vi "myRIO_BRig_Host_parse_dataTrial__read__compare.vi"(8 "input_arrayCtrl":i32[][](array[numeric]), 9 "input_idxCtrl":i32, 10 "input_arraySample":i32[][](array[numeric]), 11 "input_idxSample":i32) -> (2 "output_arraySample":i32[][](array[numeric]), 3 "output_idxSample":i32)   [LabVIEW 2014]
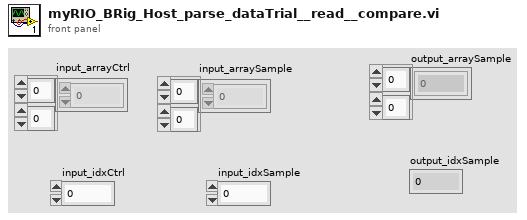
[diagram p1: front panel]
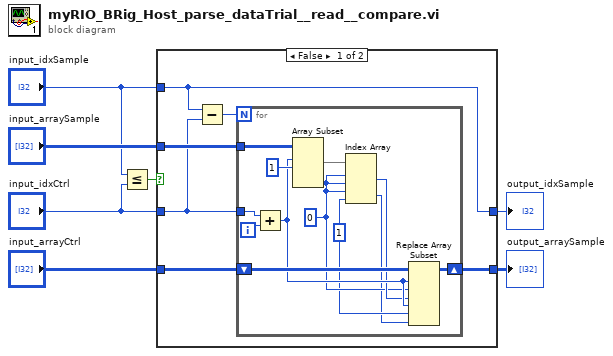
[diagram p0: block diagram]
diagram:
  n1 = Less Or Equal?(x="input_idxSample", y="input_idxCtrl") -> (x <= y?=w7:bool)
  n2 = case shown="False" w7 {
    tunnel: "input_arrayCtrl" -> [w11 w27]
    tunnel: [w10 w27] -> w5
    tunnel: "input_idxCtrl" -> [w9 w26]
    tunnel: [w12 w26] -> w3
    tunnel: "input_arraySample" -> [w13 _]
    tunnel: "input_idxSample" -> [w12 _]
    frame False {
      n3 = Subtract(x=w12, y=w9) -> (x-y=w8:i32)
      n4 = for {
        N: w8 -> [_]
        tunnel: w13 -> [w25]
        shift-right: [w23] -> w10
        shift-left: w11 -> [w24]
        tunnel: w9 -> [w22]
        i -> [w21]
        w15 = 1 ("disabled index (col)")
        w16 = 0 ("index (row)")
        n5 = Add(x=w22, y=w21) -> (x+y=w18:i32)
        n6 = Array Subset(array=w25, index (row)=w18, length (row)=1 ("length")) -> (w19:i32[][])  [unwired: 2 in]
        n7 = Index Array(array=w19, index (row) #1=w16, index (col) #1=w16, index (row) #2=w16, index (col) #2=w15) -> (element #1=w17:i32, element #2=w14:i32)
        n8 = Replace Array Subset(array=w24, new element #1=w17, index (row) #1=w18, index (col) #1=w16, new element #2=w14, index (row) #2=w18, index (col) #2=w15) -> (w23:i32[][])
      }
    }
    frame True {
    }
  }
  "output_arraySample" <- w5
  "output_idxSample" <- w3
